vi "save_template_as.vi"() -> ()   [LabVIEW 2015]
uses:
  lv-bin-template/public/_subvis/generate_error.vi
  lv-bin-template/lv-bin-template.lvlib
panel:
  out "error out":errorcluster
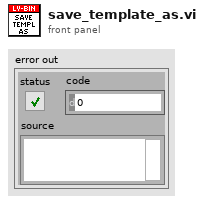
[diagram p1: front panel]
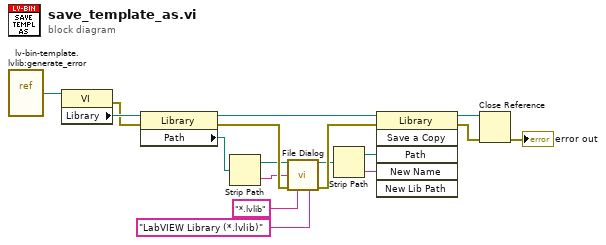
[diagram p0: block diagram]
diagram:
  n1 = vi-ref "lv-bin-template.lvlib:generate_error.vi"() -> (w1:refnum<vi>)
  n2 = property class="VI"(reference=w1) -> (error out=w4:errorcluster, "Library"=w5:refnum<vi>)  [unwired: 1 in, 1 out]
  n3 = property class="Library"(reference=w5, error in=w4) -> (reference out=w3:refnum<vi>, error out=w17:errorcluster, "Path"=w2:path)
  n4 = Strip Path(path=w2) -> (stripped path=w6:path, name=w7:string)
  n5 = call "File Dialog"("start path"=w6, "default name"=w7, "error in"=w17, "pattern (all files)"="*.lvlib", "pattern label"="LabVIEW Library (*.lvlib)") -> ("selected path"=w12:path, "error out"=w16:errorcluster)  [unwired: 7 in, 2 out]
  n6 = Strip Path(path=w12) -> (stripped path=w11:path, name=w10:string)
  n7 = invoke class="Library" method="Save a Copy"(reference=w3, error in=w16, "Path"=w11, "New Name"=w10) -> (reference out=w15:refnum<vi>, error out=w14:errorcluster)  [unwired: 2 in, 4 out]
  n8 = Close Reference(reference=w15, error in (no error)=w14) -> (error out=→"error out":errorcluster)
